vi "Proj temp.vi"() -> ()   [LabVIEW 2018]
panel:
  in  "Boolean":bool
  in  "Temperature F":dbl(slide) scale=-100.0..100.0
  out "Thermometer C":dbl(slide) scale=-100.0..100.0
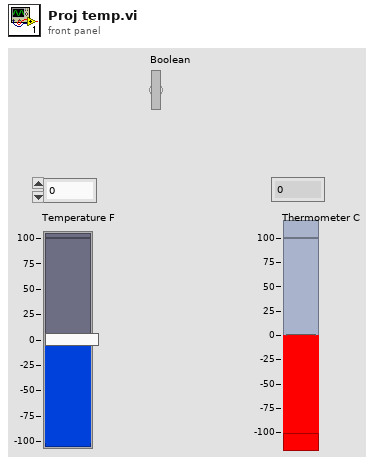
[diagram p1: front panel]
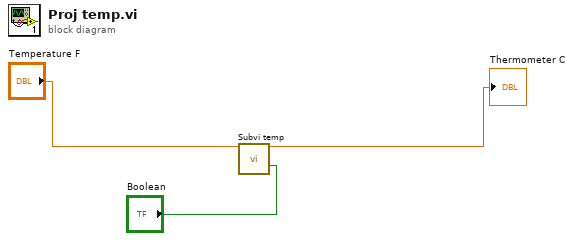
[diagram p0: block diagram]
diagram:
  n1 = call "Subvi temp.vi"("Temperature F"="Temperature F", "Boolean"="Boolean") -> ("Numeric"=→"Thermometer C":dbl)  [unwired: 13 in]
